vi "PH_Beckhoff_StepMot.get Information.vi"(0 "VI in":refnum<vi>, 5 "error in":errorcluster) -> (14 "VI out":refnum<vi>, 19 "error out":errorcluster)   [LabVIEW 2014, in "PH_Beckhoff_StepMot.lvlib"]
uses:
  PH_Beckhoff_StepMot.lvlib
  instr.lib/Beckhoff/Beckhoff - Driver np.lvlib
  PH_Beckhoff/PH_Beckhoff.lvlib
  PH_Basics/PH_Stepmotor_BaseClass/PH_Stepmotor_BaseClass.lvlib
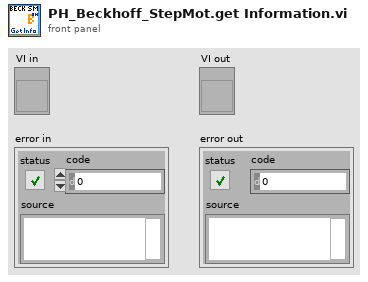
[diagram p1: front panel]
types:
  T1 = typedef "PH_Stepmotor_BaseClass.lvlib/PH_Stepmotor_BaseClass.i attribute.ctl" = cluster{"Device Error":errorcluster, "Axes PSDB Thread":cluster{"Ref":refnum<vi>, "Q-Ref":refnum<queue>, "Data Status":T2}, "Axes":T3[], "Axes PSDB Infos":cluster{"GUI Name":string, "PSDB Instance ID":i32, "PSDB Status Service ID":i32, "Axis":i32, "Class":string}[], "GUI Refs":T8}
  T2 = typedef "PH_PSDBWriter.lvlib/PH_PSDBWriter.Data Status.ctl" = i16
  T3 = typedef "PH_Stepmotor_BaseClass.lvlib/PH_Stepmotor_BaseClass.Axis Attributes.ctl" = cluster{"Settings":T4, "Endswitch?":bool, "DIM Service IDs":T6, "Activity":T7, "Configured?":bool, "Position":cluster{"Current":i32, "Target":i32}, "Position to set":cluster{"New?":bool, "Wanted":i32}, "Stop?":bool, "Reset?":bool, "Move?":bool, "Nothing connected?":bool}
  T4 = typedef "PH_Stepmotor_BaseClass.lvlib/PH_Stepmotor_BaseClass.Axis Settings.ctl" = cluster{"Sign change":bool, "Width":dbl, "Calibration":dbl, "Unit":string, "Motor Type":T5, "Unit Width":string, "Unit CF":string}
  T5 = typedef "PH_Stepmotor_BaseClass.lvlib/PH_Stepmotor_BaseClass.Motor Type.ctl" = enum16{"Unspecific", "OWIS 49.120.2633", "OWIS 49.060.1033", "OWIS 43.040.2558", "Diamond Motion 2200 series", "OWIS 49.120.266B.MV6", "Calorimeter", "Linear Stage 1", "MICOS VT-80", "MICOS VT-80 S", "Standa Rotstage nt0.95A", "PUF RA 320.200", "PUF RA 800.200", "PUF RA 800.400", "PUF RA 400.50", "1324.nn.800.50", "1324.n9c.800.50", "1324.nn.320.200", "1324.nn.400.200", "1324.nn.800.200", "1324.nn.400.50", "1324.8c9c.800.50", "1324.8c9c.400.200"}
  T6 = typedef "PH_Stepmotor_BaseClass.lvlib/PH_Stepmotor_BaseClass.Axis DIM Service IDs.ctl" = cluster{"Settings":i32, "Information":i32}
  T7 = typedef "PH_Stepmotor_BaseClass.lvlib/PH_Stepmotor_BaseClass.Axis Activity.ctl" = enum16{"No Information", "stopped", "running", "Failure", "Alarm", "stopped at backward ES", "stopped at foreward ES"}
  T8 = typedef "PH_Stepmotor_BaseClass.lvlib/PH_Stepmotor_BaseClass.GUI Refs.ctl" = cluster{"Axes Configuration":refnum<vi>, "Device Error":refnum<vi>, "Axes PSDB Infos":refnum<vi>}
  T9 = typedef "PH_Beckhoff_StepMot.lvlib/PH_Beckhoff_StepMot.i attribute.ctl" = cluster{"Axes Settings":T10[], "GUI Refs":cluster{"Axes Settings":refnum<vi>, "Stati":refnum<vi>}, "Get Beckhoff Settings":bool}
  T10 = typedef "PH_Beckhoff_StepMot.lvlib/PH_Beckhoff_StepMot.Axis Cluster.ctl" = cluster{"Step Motor Configuration":T11, "To set?":bool, "Endswitch inverted?":bool}
  T11 = typedef "Beckhoff - Driver np.lvlib/Beckhoff.Step Motor - Motor Configuration.ctl" = cluster{"Feature Register":T12, "I max A [mA]":dbl, "I max B [mA]":dbl, "v min":u32, "v max":u32, "a max":u32, "I hold [%]":u32, "Steps/qp":u32, "Feature Register 2":T13}
  T12 = typedef "Beckhoff - Driver np.lvlib/Beckhoff.Step Motor - Feature Register 1.ctl" = cluster{"en Auto Start":bool, "en Auto Stop":bool, "dis Wd Timer":bool, "OP Mode 1":bool, "OP Mode 2":bool, "Ramp Type":bool, "inv Pos Feedback":bool, "en User Cur Table":bool, "en Latch Evt Clr Pos":bool, "en Multi Latch Vals":bool, "en Sign Disp*":bool, "Feedback Type*":bool, "en neg Gate Lock*":bool, "en pos Gate Lock*":bool, "dis Enc Fltr*":bool, "en Counter Mode*":bool}
  T13 = typedef "Beckhoff - Driver np.lvlib/Beckhoff.Step Motor - Feature Register 2.ctl" = cluster{"rev Homing Dir":bool, "en Decac Ramp":bool, "Latch Reg Pos":bool, "Show Idle":bool, "dis Ref Input 1":bool, "dis Ref Input 2":bool, "en ext Auto Start":bool, "N/A":bool, "N/A":bool, "N/A":bool, "N/A":bool, "N/A":bool, "en Clr Proc Data":bool, "en Man Ecl Tolerce*":bool, "rev Dig Input 1":bool, "rev Dig Input 2":bool}
  T14 = typedef "PH_Beckhoff.lvlib/PH_Beckhoff.i attribute.ctl" = cluster{"GUI Refs":T15, "operation?":bool, "Default Prdc Interval":i32, "Connection":T16, "AMS Net ID":T17, "Klemmencluster: # of":T18, "Values":T19, "IP":string, "Description":string, "configured?":bool, "Change Manager":cluster{"Detemination wanted?":bool, "Values changed at":cluster{"Sonderklemmen Inputs":i32[], "Analog Inputs":i32[], "Analog Outputs":i32[], "Digital Inputs":i32[], "Digital Outputs":i32[]}}, "Difference to handle an analog input as change":u32}
  T15 = typedef "PH_Beckhoff.lvlib/PH_Beckhoff.GUI Refs.ctl" = cluster{"ADS Error":refnum<vi>, "Values":refnum<vi>, "configured?":refnum<vi>, "Connection":refnum<vi>, "IP":refnum<vi>, "Prdc Int [ms]":refnum<vi>}
  T16 = typedef "PH_Beckhoff.lvlib/PH_Beckhoff.Connectivity.ctl" = cluster{"DLL?":bool, "Port?":bool, "Client?":bool, "Ping?":bool, "unsuccessful Pings":u32}
  T17 = typedef "Beckhoff - Driver np.lvlib/Beckhoff Access.ctl" = cluster{"DLL path":path, "AMS Net ID":cluster{"1st # of IP":u8, "2nd # of IP":u8, "3rd # of IP":u8, "4th # of IP":u8, "In Port":u8, "Out Port":u8}}
  T18 = typedef "Beckhoff - Driver np.lvlib/Klemmendeclarer.ctl" = cluster{"Offset due to Sonderklemms":u32, "analog Inputs":u32, "analog Outputs":u32, "digital Input Bits":u32, "digital Output Bits":u32}
  T19 = typedef "PH_Beckhoff.lvlib/PH_Beckhoff.Values.ctl" = cluster{"Sonderklemmen Inputs":T20, "Analog Inputs":T21, "Analog Outputs":T23, "Digital Inputs":T24, "Digital Outputs":T25}
  T20 = typedef "PH_Beckhoff.lvlib/PH_Beckhoff.Sonderklemmen Inputs.ctl" = cluster{"Total Length":u32, "Name":string, "Value":u64, "Quality":bool, "Service ID":i32, "Offset":u32, "Length":u32}[]
  T21 = typedef "PH_Beckhoff.lvlib/PH_Beckhoff.Analog Inputs.ctl" = cluster{"Name":string, "Value":u32, "Quality":bool, "Service ID":i32, "Sca Type":T22}[]
  T22 = typedef "PH_Beckhoff.lvlib/PH_Beckhoff.Scaling Type.ctl" = enum16{"none", "0 ... 15 Bit -> 0 ... 5", "0 ... 15 Bit -> 0 ... 10", "0 ... 15 Bit -> 0 ... 25", "0 ... 15 Bit -> 4 ... 20", "0 ... 15 Bit -> 0 ... 1", "0 ... 15 Bit -> 0 ... 20000", "0 ... 15 Bit -> 0 ... 24000"}
  T23 = typedef "PH_Beckhoff.lvlib/PH_Beckhoff.Analog Outputs.ctl" = cluster{"Name":string, "Value":u32, "Quality":bool, "Wanted Value":u32, "Service ID":i32, "Sca Type":T22}[]
  T24 = typedef "PH_Beckhoff.lvlib/PH_Beckhoff.Digital Inputs.ctl" = cluster{"Name":string, "Value":bool, "Quality":bool, "Service ID":i32, "inverted?":bool}[]
  T25 = typedef "PH_Beckhoff.lvlib/PH_Beckhoff.Digital Outputs.ctl" = cluster{"Name":string, "Value":bool, "Quality":bool, "Wanted Value":bool, "Service ID":i32, "inverted?":bool}[]
  T26 = typedef "Beckhoff - Driver np.lvlib/Beckhoff.Step Motor - Status.ctl" = cluster{"Byte":T27, "Word":T28}
  T27 = typedef "Beckhoff - Driver np.lvlib/Beckhoff.Step Motor - Status Byte.ctl" = cluster{"Ready":bool, "Load Angle 1":bool, "Load Angle 2":bool, "Load Angle 3":bool, "Idle":bool, "Warning":bool, "Error":bool, "RegAccess":bool}
  T28 = typedef "Beckhoff - Driver np.lvlib/Beckhoff.Step Motor - Status Word.ctl" = cluster{"Input 1":bool, "Input 2":bool, "Set Pos Ready":bool, "Target reached":bool, "Latch valid":bool, "Latch Data InByte 2,3":bool, "Latch Data toggled":bool, "Eencoder disabled":bool, "Over temperature":bool, "Under voltage":bool, "Open load Br A":bool, "Open load Br B":bool, "Over current Br A":bool, "Over current Br B":bool, "No control Power":bool, "Config Error":bool}
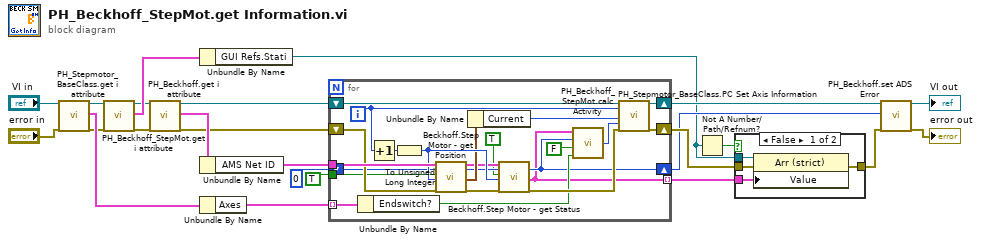
[diagram p0: block diagram]
diagram:
  n1 = call "PH_Stepmotor_BaseClass.get i attribute.vi"("i ref in"="VI in", "error in (no error)"="error in") -> ("i ref out"=w8:refnum<vi>, "i attribute"=w17:T1, "error out"=w7:errorcluster)  [unwired: 15 in]
  n2 = call "PH_Beckhoff_StepMot.get i attribute.vi"("i ref in"=w8, "error in (no error)"=w7) -> ("i ref out"=w10:refnum<vi>, "i attribute"=w18:T9, "error out"=w9:errorcluster)  [unwired: 15 in]
  n3 = call "PH_Beckhoff.get i attribute.vi"("i ref in"=w10, "error in (no error)"=w9) -> ("i ref out"=w22:refnum<vi>, "i attribute"=w21:T14, "error out"=w19:errorcluster)  [unwired: 15 in]
  n4 = Unbundle By Name(w18) -> ("GUI Refs.Stati"=w1:refnum<vi>)
  n5 = Unbundle By Name(w21) -> ("AMS Net ID"=w20:T17)
  n6 = Unbundle By Name(w17) -> ("Axes"=w16:T3[])
  n7 = for {
    tunnel: w20 -> [w47]
    shift-right: [w40] -> w15
    shift-left: w22 -> [w37]
    shift-right: [w39] -> w14
    shift-left: w19 -> [w46]
    shift-right: [w27] -> w13
    shift-left: 0 ("ADS Error out") -> [w43]
    tunnel: w16 -> [w42] mode=indexing
    tunnel: TRUE ("Read?") -> [w41]
    tunnel: [w26] -> w3 mode=indexing
    i -> [w38]
    n8 = Unbundle By Name(w42) -> ("Endswitch?"=w28:bool)
    n9 = Increment(x=w38) -> (x+1=w45:i32)
    n10 = To Unsigned Long Integer(number=w45) -> (unsigned 32bit integer=w44:u32)
    n11 = call "Beckhoff.Step Motor - get Position.vi"("AMS Net ID in"=w47, "ADS Error in (0)"=w43, "Read?"=w41, "# of Klemme [1, ...]"=w44, "error in (no error)"=w46) -> ("AMS Net ID out"=w35:T17, "ADS Error out"=w34:i32, "Position"=w36:cluster{"Target":i32, "Current":i32}, "error out"=w33:errorcluster)  [unwired: 10 in, 1 out]
    n12 = Unbundle By Name(w36) -> ("Current"=w30:i32)
    n13 = call "Beckhoff.Step Motor - get Status.vi"("AMS Net ID in"=w35, "ADS Error in (0)"=w34, "Read?"=TRUE, "# of Klemme [1, ...]"=w44, "error in (no error)"=w33) -> ("ADS Error out"=w27:i32, "Status"=w26:T26, "error out"=w31:errorcluster)  [unwired: 10 in, 2 out]
    n14 = call "PH_Beckhoff_StepMot.calc Activity.vi"("Endswitch?"=w28, "Moving"=FALSE, "ADS Error in"=w27, "Status"=w26) -> ("Axis Activity"=w29:T7)
    n15 = call "PH_Stepmotor_BaseClass.PC Set Axis Information.vi"("i ref in"=w37, "axis"=w38, "Current Position (Steps)"=w30, "Axis Activity"=w29, "error in (no error)"=w31) -> ("i ref out"=w40:refnum<vi>, "error out"=w39:errorcluster)  [unwired: 13 in]
  }
  n16 = Not A Number/Path/Refnum?(number/path/refnum=w1) -> (NaN/Path/Refnum?=w2:bool)
  n17 = case shown="False" w2 {
    tunnel: w14 -> [w51 w52]
    tunnel: [w50 w52] -> w4
    tunnel: w1 -> [w49 _]
    tunnel: w3 -> [w48 _]
    frame False {
      n18 = property class="Arr (strict)"(reference=w49, error in=w51, "Value"=w48) -> (error out=w50:errorcluster)  [unwired: 1 out]
    }
    frame True {
    }
  }
  n19 = call "PH_Beckhoff.set ADS Error.vi"("i ref in"=w15, "ADS Error"=w13, "error in"=w4) -> ("i ref out"=→"VI out":refnum<vi>, "error out"=→"error out":errorcluster)  [unwired: 15 in]
